vi "getErrorInfo.vi"(8 "error in (no error)":errorcluster, 11 "Logger in":refnum<class "Logger.lvclass">) -> (0 "error out":errorcluster, 2 "infoErr":string, 3 "Logger out":refnum<class "Logger.lvclass">)   [LabVIEW 2018, in "Logger.lvclass"]
doc: "Get the error information in the error in terminal."
uses:
  Logger.lvclass
  <vilib>/Utility/error.llb/DialogType.ctl
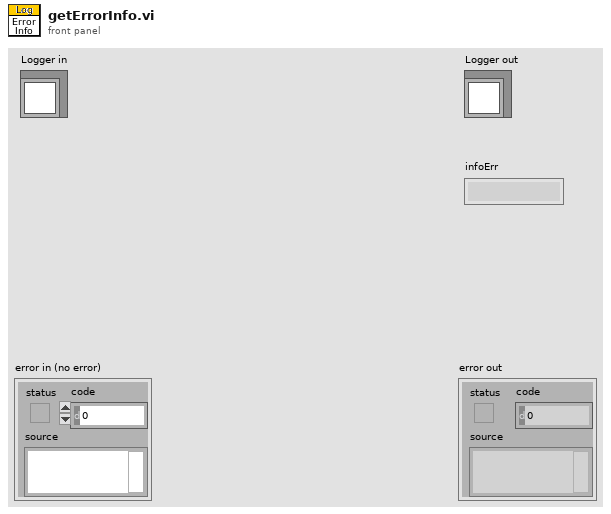
[diagram p1: front panel]
types:
  T1 = typedef "DialogType.ctl" = u16
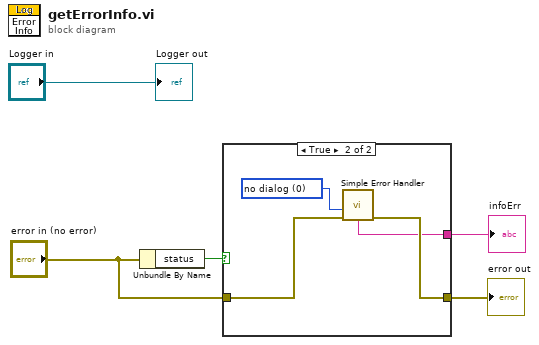
[diagram p0: block diagram]
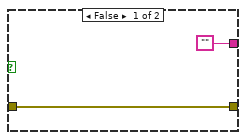
[diagram p2: hidden frame]
diagram:
  n1 = Unbundle By Name("error in (no error)") -> ("status"=w4:bool)
  n2 = case shown="True" w4 {
    tunnel: "error in (no error)" -> [w6 w10]
    tunnel: ["" w8] -> w3
    tunnel: [w6 w9] -> w1
    frame False {
    }
    frame True {
      w11 = T1 0 items=["no dialog", "OK message", "continue or stop message", "OK message + warnings", "continue/stop + warnings"] ("type of dialog (OK msg:1)")
      n3 = call <vilib>:"Simple Error Handler.vi"("type of dialog (OK msg:1)"=w11, "error in (no error)"=w10) -> ("error out"=w9:errorcluster, "message"=w8:string)  [unwired: 3 in, 3 out]
    }
  }
  "error out" <- w1
  "infoErr" <- w3
  "Logger out" <- "Logger in"
